vi "Device Params 2 Config XML File.vi"(5 "Data Acquisition Parameters":T1={"Experiment Type"=enum."PID Sample", "Experiment Name"="", "Operator Name"="", "Notes"="", "TDMS File Path"=path "", "Data Acquisition State"=FALSE, "PID Voltage Sweep"={"Voltage Step (V)"=1.0, "Voltage Range (V)"={10, 20}, "Time Step (s)"=5.0, "Voltage Step Direction"=enum."Low 2 High"}, "MFC Challenge Profile - Heaviside Step"={"Valve Open Duration"=20, "MFC Flow Rate"=100.0, "Valve Open Repeats"=50, "Valve Open Start"=1}, "MFC Challenge Profile"=enum."Heaviside", "MFC Challenge Profile - Staircase"={"Step Time Duration"=1, "Step Flow Rate"=0.0, "Steps"=1, "Valve Open Start"=1, "Recovery"=FALSE, "Repeats"=1}} {"MFC Challenge Profile - Staircase"."Repeats" min=1 max=1000 step=1; "MFC Challenge Profile - Staircase"."Valve Open Start" min=1 max=1000 step=1; "MFC Challenge Profile - Staircase"."Steps" min=1 max=1000 step=1; "MFC Challenge Profile - Staircase"."Step Flow Rate" min=0.0 max=200.0 scale=0.0..200.0; "MFC Challenge Profile - Staircase"."Step Time Duration" min=1 max=1000 step=1; "MFC Challenge Profile - Heaviside Step"."Valve Open Start" min=1 max=1000 step=1; "MFC Challenge Profile - Heaviside Step"."Valve Open Repeats" min=1 max=1000 step=1; "MFC Challenge Profile - Heaviside Step"."MFC Flow Rate" min=0.0 max=200.0 scale=0.0..200.0; "MFC Challenge Profile - Heaviside Step"."Valve Open Duration" min=1 max=1000 step=1; "PID Voltage Sweep"."Voltage Range (V)" scale=0.0..500.0}, 7 "error in":errorcluster, 8 "Device Connections":T7={"Detector"={"Detector Type"=enum."INL PID", "Connection"=FALSE, "B-M PID"={"AI DAQmx channel"=""}, "INL PID Connections"={"PIDs"=1, "Integrator DAQ Channels 1"={"V0"="cDAQ1Mod1/ai0", "S1"="cDAQ1Mod5/port0/line4", "S2"="cDAQ1Mod5/ctr0"}, "Integrator DAQ Channels 2"={"V0"="cDAQ1Mod1/ai0", "S1"="cDAQ1Mod5/port0/line4", "S2"="cDAQ1Mod5/ctr0"}}}, "Power Supply"={"Type"=enum."Stanford Research PS350", "Connection"=FALSE, "VISA resource name"=""}, "Mass Flow Controller"={"Type"=enum."Aalborg GFC17", "Connection"=FALSE, "Aalborg GFC17"={"flow rate setpoint channel"="cDAQ1Mod3/ao0", "flow rate reading channel"="cDAQ1Mod1/ai4", "valve channel"="cDAQ1Mod3/ao1"}}, "Valve Controller"={"Type"=enum."SMC - INL", "Connection"=FALSE, "SMC - INL"={"VISA resource name"="COM3"}}, "Multimeter"={"Multimeter Type"=enum."Agilent 3458A", "Connection"=FALSE, "VISA resource name"=""}, "Vapour Generator"={"Type"=enum."Owlstone GEN-SYS", "Connection"=FALSE, "Owlstone Gen-SYS"={"GEN-SYS VISA resource name"="", "OVG-4"={"Flow Address"=2, "Temp Address"=1}, "OHG-4"={"Flow Address"=2, "Easydew VISA resource name"=""}}}} {"Detector"."INL PID Connections"."PIDs" min=1 max=2 step=1}, 9 "Device Settings":T17={"PID"={"B-M PID"={"Detector Sampling Frequency"=0.0}, "INL PID"={"Sampling Frequency"=0.5, "Integration Time"=50.0, "Integration Periods"=50, "Grid Voltage"=50.0}}, "Power Supply"={"Source Value"=0.0, "Source Value Units"=enum."volts", "Source Mode"=enum."Volts", "Limits"={"Voltage Limit"=0.0, "Voltage Limit Units"=enum."volts", "Current Limit"=0.0, "Current Limit Units"=enum."amps", "Voltage Trip/Cmpl"=0.0, "Voltage Trip/Cmpl Units"=enum."volts", "Current Trip/Cmpl"=0.0, "Current Trip/Cmpl Units"=enum."amps"}, "Output"=FALSE}, "Mass Flow Controller"={"MFC Flow Rate"=0.0, "MFC Valve Status"=enum."Open"}, "Valve Controller"={"Valve Assembly"={"Valve 1"=0, "Valve 2"=0, "Valve 3"=0, "Valve 4"=0, "Valve 5"=0}}, "Multimeter"={"Agilent 3458A"={"Measurement Configuration"={"Function"=enum."2-Wire Resistance", " Manual Resolution"=enum."6.5", "Frequency Source"=enum."AC Voltage", "Auto Range"=enum."ON"}, "Measurement Integration"={"Power Line Cycles"=0.0}}}, "Vapour Generator"={"Owlstone Permeation Tube"={"Tube"=enum."Isobutylene 27 Nov 2012", "Molecular Weight"=0.0, "Calibration Temperature\n(Celcius)"=0, "Permeation Rate \n(ng/min)"=0}, "Owlstone GEN-SYS Setpoints"={"OVG-4"={"Oven Temperature"=0, "Sample Flow Rate"=0, "Split Flow Status"=0, "Split Flow Rate"=0}, "OHG-4"={"Wet Air Flow"=0}}}} {"Vapour Generator"."Owlstone GEN-SYS Setpoints"."OHG-4"."Wet Air Flow" min=300 max=3000 scale=300.0..3000.0; "Vapour Generator"."Owlstone GEN-SYS Setpoints"."OVG-4"."Split Flow Status" items=["Closed", "Open"]; "Vapour Generator"."Owlstone GEN-SYS Setpoints"."OVG-4"."Split Flow Rate" min=300 max=3000 scale=50.0..3000.0; "Vapour Generator"."Owlstone GEN-SYS Setpoints"."OVG-4"."Sample Flow Rate" min=50 max=500 scale=50.0..500.0; "Vapour Generator"."Owlstone GEN-SYS Setpoints"."OVG-4"."Oven Temperature" min=25 max=100 scale=25.0..100.0; "Vapour Generator"."Owlstone Permeation Tube"."Molecular Weight" min=0.0 format="%#_3g"; "Vapour Generator"."Owlstone Permeation Tube"."Permeation Rate \n(ng/min)" min=0; "Vapour Generator"."Owlstone Permeation Tube"."Calibration Temperature\n(Celcius)" min=0; "Valve Controller"."Valve Assembly"."Valve 5" items=["Closed", "Open"]; "Valve Controller"."Valve Assembly"."Valve 4" items=["Closed", "Open"]; "Valve Controller"."Valve Assembly"."Valve 3" items=["Closed", "Open"]; "Valve Controller"."Valve Assembly"."Valve 2" items=["Closed", "Open"]; "Valve Controller"."Valve Assembly"."Valve 1" items=["Closed", "Open"]}, 10 "Configuration in":refnum<class "Configuration.lvclass">) -> (0 "error out":errorcluster, 3 "Configuration out":refnum<class "Configuration.lvclass">)   [LabVIEW 2011]
uses:
  Modules/File/Configuration/Configuration.lvclass
  Controls/Device Settings.ctl
  Modules/Hardware/Baseline Mocon piD-Tech plus/Settings.ctl
  Modules/Hardware/INL PID/Settings.ctl
  Modules/Hardware/Power Supply/Source Units.ctl
  Modules/Hardware/Power Supply/Source Mode.ctl
  Modules/Hardware/Power Supply/Protection Limits.ctl
  Modules/Hardware/Power Supply/Voltage Units.ctl
  Modules/Hardware/Power Supply/Current Units.ctl
  Modules/Hardware/Mass Flow Controller/Valve Status.ctl
  Modules/Hardware/Valve Controller/Valve Assembly.ctl
  Modules/Hardware/Valve Controller/Status.ctl
  Modules/Hardware/Agilent 3458A/Measurement Configuration.ctl
  Modules/Hardware/Agilent 3458A/Measurement Integration.ctl
  Modules/Hardware/Owlstone GEN-SYS/Permeation Tube.ctl
  Modules/Hardware/Owlstone GEN-SYS/Permeation Tube Gas.ctl
  Modules/Hardware/Owlstone GEN-SYS/Gen-Sys Setpoints.ctl
  Controls/Device Connections.ctl
  Controls/Detector Type.ctl
  Modules/Hardware/Baseline Mocon piD-Tech plus/Connections.ctl
  Controls/INL PID Connections.ctl
  Modules/Hardware/INL PID/Integrator DAQmx Channels.ctl
  Modules/Hardware/Aalborg GFC17/Aalborg GFC17 Connections.ctl
  Controls/Valve Type.ctl
  Controls/Multimeter Type.ctl
  Controls/Vapour Generator Type.ctl
  Modules/Hardware/Owlstone GEN-SYS/GEN-SYS Connections.ctl
  Controls/Data Acquisition Parameters.ctl
  Controls/DAQ Type.ctl
  Controls/PID Voltage Seep Settings.ctl
  Controls/MFC Challenge Profile - Heaviside Step.ctl
  Controls/MFC Challen Profile Type.ctl
  Controls/MFC Challenge Profile - Staircase.ctl
  Modules/Hardware/Power Supply/Power Supply.lvclass
  Modules/Hardware/Mass Flow Controller/Mass Flow Controller.lvclass
  Modules/Hardware/INL PID/INL PID.lvclass
  Modules/Hardware/Valve Controller/Valve Controller.lvclass
  Modules/Hardware/Aalborg GFC17/Aalborg GFC17.lvclass
  Modules/Hardware/Agilent 3458A/Agilent 3458A.lvclass
  Modules/Hardware/Owlstone GEN-SYS/Owlstone GEN-SYS.lvclass
  Modules/Hardware/Baseline Mocon piD-Tech plus/Baseline Mocon piD-Tech plus.lvclass
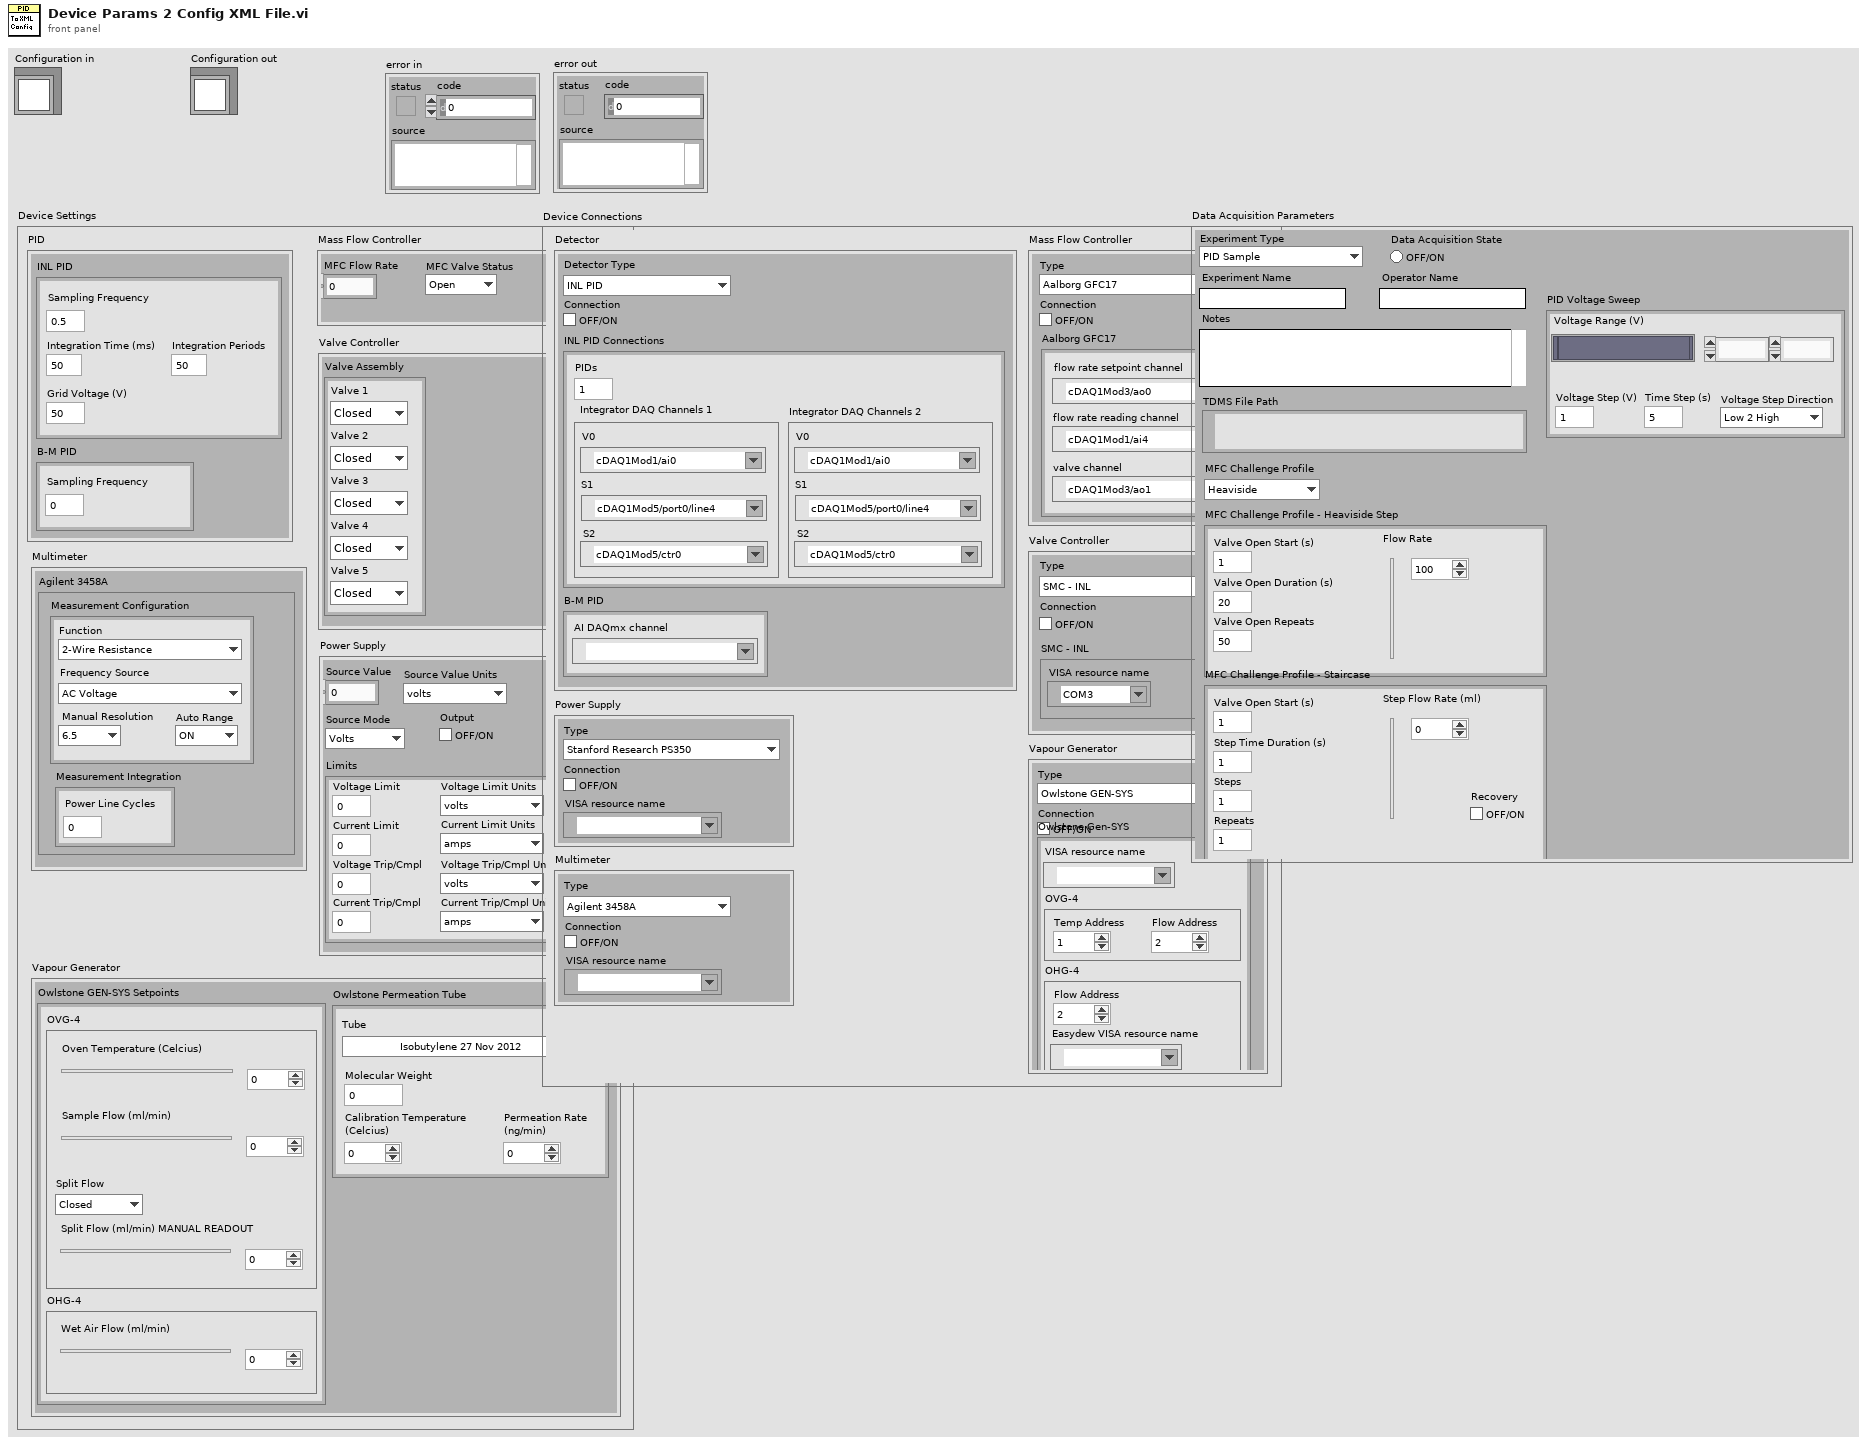
[diagram p1: front panel]
types:
  T1 = typedef "Data Acquisition Parameters.ctl" = cluster{"Experiment Type":T2, "Experiment Name":string, "Operator Name":string, "Notes":string, "TDMS File Path":path, "Data Acquisition State":bool, "PID Voltage Sweep":T3, "MFC Challenge Profile - Heaviside Step":T4, "MFC Challenge Profile":T5, "MFC Challenge Profile - Staircase":T6}
  T2 = typedef "DAQ Type.ctl" = enum16{"PID Sample", "PID with PS Challenge", "PID with MFC Challenge", "Multimeter Sample", "Multimeter with MFC Challenge"}
  T3 = typedef "PID Voltage Seep Settings.ctl" = cluster{"Voltage Step (V)":dbl, "Voltage Range (V)":cluster{u16, u16}, "Time Step (s)":dbl, "Voltage Step Direction":enum16{"High 2 Low", "Low 2 High"}}
  T4 = typedef "MFC Challenge Profile - Heaviside Step.ctl" = cluster{"Valve Open Duration":u16, "MFC Flow Rate":dbl, "Valve Open Repeats":u16, "Valve Open Start":u16}
  T5 = typedef "MFC Challen Profile Type.ctl" = enum16{"Heaviside", "Staircase"}
  T6 = typedef "MFC Challenge Profile - Staircase.ctl" = cluster{"Step Time Duration":u16, "Step Flow Rate":dbl, "Steps":u16, "Valve Open Start":u16, "Recovery":bool, "Repeats":u16}
  T7 = typedef "Device Connections.ctl" = cluster{"Detector":cluster{"Detector Type":T8, "Connection":bool, "B-M PID":T9, "INL PID Connections":T10}, "Power Supply":cluster{"Type":enum16{"Stanford Research PS350", "Keithley 2400"}, "Connection":bool, "VISA resource name":refnum<visa-resource-name>}, "Mass Flow Controller":cluster{"Type":enum16{"Aalborg GFC17"}, "Connection":bool, "Aalborg GFC17":T12}, "Valve Controller":cluster{"Type":T13, "Connection":bool, "SMC - INL":cluster{"VISA resource name":refnum<visa-resource-name>}}, "Multimeter":cluster{"Multimeter Type":T14, "Connection":bool, "VISA resource name":refnum<visa-resource-name>}, "Vapour Generator":cluster{"Type":T15, "Connection":bool, "Owlstone Gen-SYS":T16}}
  T8 = typedef "Detector Type.ctl" = enum16{"INL PID", "Baseline-Mocon piD-TECH plus"}
  T9 = typedef "Baseline Mocon piD-Tech plus.lvclass/Connections.ctl" = cluster{"AI DAQmx channel":tag}
  T10 = typedef "INL PID Connections.ctl" = cluster{"PIDs":u8, "Integrator DAQ Channels 1":T11, "Integrator DAQ Channels 2":T11}
  T11 = typedef "INL PID.lvclass/Integrator DAQmx Channels.ctl" = cluster{"V0":tag, "S1":tag, "S2":tag}
  T12 = typedef "Aalborg GFC17.lvclass/Aalborg GFC17 Connections.ctl" = cluster{"flow rate setpoint channel":tag, "flow rate reading channel":tag, "valve channel":tag}
  T13 = typedef "Valve Type.ctl" = enum16{"SMC - INL"}
  T14 = typedef "Multimeter Type.ctl" = enum16{"Agilent 3458A"}
  T15 = typedef "Vapour Generator Type.ctl" = enum16{"Owlstone GEN-SYS"}
  T16 = typedef "Owlstone GEN-SYS.lvclass/GEN-SYS Connections.ctl" = cluster{"GEN-SYS VISA resource name":refnum<visa-resource-name>, "OVG-4":cluster{"Flow Address":u8, "Temp Address":u8}, "OHG-4":cluster{"Flow Address":u8, "Easydew VISA resource name":refnum<visa-resource-name>}}
  T17 = typedef "Device Settings.ctl" = cluster{"PID":cluster{"B-M PID":T18, "INL PID":T19}, "Power Supply":cluster{"Source Value":dbl, "Source Value Units":T20, "Source Mode":T21, "Limits":T22, "Output":bool}, "Mass Flow Controller":cluster{"MFC Flow Rate":dbl, "MFC Valve Status":T25}, "Valve Controller":cluster{"Valve Assembly":T26}, "Multimeter":cluster{"Agilent 3458A":cluster{"Measurement Configuration":T28, "Measurement Integration":T29}}, "Vapour Generator":cluster{"Owlstone Permeation Tube":T30, "Owlstone GEN-SYS Setpoints":T32}}
  T18 = typedef "Baseline Mocon piD-Tech plus.lvclass/Settings.ctl" = cluster{"Detector Sampling Frequency":dbl}
  T19 = typedef "INL PID.lvclass/Settings.ctl" = cluster{"Sampling Frequency":dbl, "Integration Time":dbl, "Integration Periods":u8, "Grid Voltage":dbl}
  T20 = typedef "Power Supply.lvclass/Source Units.ctl" = enum16{"volts", "millivolts", "microvolts", "amps", "milliamps", "microamps", "nanoamps"}
  T21 = typedef "Power Supply.lvclass/Source Mode.ctl" = enum16{"Volts", "Current"}
  T22 = typedef "Power Supply.lvclass/Protection Limits.ctl" = cluster{"Voltage Limit":dbl, "Voltage Limit Units":T23, "Current Limit":dbl, "Current Limit Units":T24, "Voltage Trip/Cmpl":dbl, "Voltage Trip/Cmpl Units":T23, "Current Trip/Cmpl":dbl, "Current Trip/Cmpl Units":T24}
  T23 = typedef "Power Supply.lvclass/Voltage Units.ctl" = enum16{"volts", "millivolts", "microvolts"}
  T24 = typedef "Power Supply.lvclass/Current Units.ctl" = enum16{"amps", "milliamps", "microamps", "nanoamps"}
  T25 = typedef "Mass Flow Controller.lvclass/Valve Status.ctl" = enum16{"Open", "Closed"}
  T26 = typedef "Valve Controller.lvclass/Valve Assembly.ctl" = cluster{"Valve 1":T27, "Valve 2":T27, "Valve 3":T27, "Valve 4":T27, "Valve 5":T27}
  T27 = typedef "Valve Controller.lvclass/Status.ctl" = u16
  T28 = typedef "Agilent 3458A.lvclass/Measurement Configuration.ctl" = cluster{"Function":enum16{"DC Voltage", "AC Voltage", "AC + DC Voltage", "DC Current", "AC Current", "AC + DC Current", "2-Wire Resistance", "4-Wire Resistance", "Frequency", "Period", "Direct Sampling DC", "Direct Sampling AC", "Sub-Sampling DC", "Sub-Sampling AC"}, " Manual Resolution":enum16{"4.5", "5.5", "6.5", "7.5", "8.5"}, "Frequency Source":enum16{"AC + DC Current", "AC + DC Voltage", "AC Current", "AC Voltage"}, "Auto Range":enum16{"OFF", "ON", "ONCE"}}
  T29 = typedef "Agilent 3458A.lvclass/Measurement Integration.ctl" = cluster{"Power Line Cycles":dbl}
  T30 = typedef "Owlstone GEN-SYS.lvclass/Permeation Tube.ctl" = cluster{"Tube":T31, "Molecular Weight":dbl, "Calibration Temperature\n(Celcius)":i32, "Permeation Rate \n(ng/min)":i32}
  T31 = typedef "Owlstone GEN-SYS.lvclass/Permeation Tube Gas.ctl" = enum16{"Isobutylene 27 Nov 2012", "Ammonia 29 Sep 2012", "DMMP Tube A 3 July 2014", "DMMP Tube B 3 July 2014"}
  T32 = typedef "Owlstone GEN-SYS.lvclass/Gen-Sys Setpoints.ctl" = cluster{"OVG-4":cluster{"Oven Temperature":i32, "Sample Flow Rate":i32, "Split Flow Status":u16, "Split Flow Rate":i32}, "OHG-4":cluster{"Wet Air Flow":i32}}
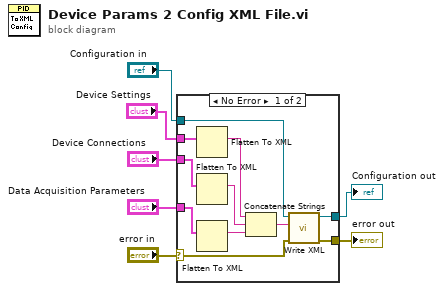
[diagram p0: block diagram]
diagram:
  n1 = case shown="No Error" "error in" {
    selector: "error in" -> [w18 w19]
    tunnel: [w10 w20] -> w7
    tunnel: "Configuration in" -> [w17 w20]
    tunnel: [w11 w19] -> w5
    tunnel: "Device Settings" -> [w16 _]
    tunnel: "Device Connections" -> [w15 _]
    tunnel: "Data Acquisition Parameters" -> [w9 _]
    frame No Error {
      n2 = Flatten To XML(anything=w16) -> (xml string=w14:string)
      n3 = Flatten To XML(anything=w15) -> (xml string=w13:string)
      n4 = Flatten To XML(anything=w9) -> (xml string=w8:string)
      n5 = Concatenate Strings(w14, w13, w8) -> (w12:string)
      n6 = call-dynamic "Write XML.vi"("error in (no error)"=w18, "String"=w12, "Configuration in"=w17) -> ("error out"=w11:errorcluster, "Configuration out"=w10:refnum<class "Configuration.lvclass">)  [unwired: 7 in]
    }
    frame Error {
    }
  }
  "Configuration out" <- w7
  "error out" <- w5
